vi "Create_SourceItem_from_Linker.vi"(8 "error in (no error)":errorcluster, 9 "Ignore unresolved dll reference (F)":bool, 10 "linkerInfo":T2) -> (0 "error out":errorcluster, 2 "valid?":bool, 3 "AB_Source out":refnum<class "AB_Source.lvclass">)   [LabVIEW 2020, in "AB_Source.lvclass"]
uses:
  <vilib>/AppBuilder/AB_Classes/Source/AB_Source.lvclass
  <vilib>/Utility/lvfile.llb/LVFileType.ctl
  <vilib>/AppBuilder/AB_Classes/Source/AB_Source.ctl
  <vilib>/AppBuilder/AB_Source_Inclusion.ctl
  <vilib>/AppBuilder/AB_Source_Properties.ctl
  <vilib>/AppBuilder/AB_Source_Property_Type.ctl
  <vilib>/AppBuilder/AB_Classes/Source/VI/AB_Source_VI.ctl
  <vilib>/AppBuilder/AB_Classes/Source/VI/AB_Source_VI.lvclass
  e:/builds/penguin/labview/branches/2020/dev/dist/vi.lib/AppBuilder/AB_Classes/Source/AB_Source.lvclass
  <vilib>/AppBuilder/AB_Classes/Source/Library/AB_Source_Library.ctl
  <vilib>/AppBuilder/AB_Classes/Source/Library/AB_Source_Library.lvclass
  <vilib>/AppBuilder/AB_Classes/Source/PackedItem/AB_Source_PackedItem.lvclass
  <vilib>/Utility/lvfile.llb/NI_FileType.lvlib
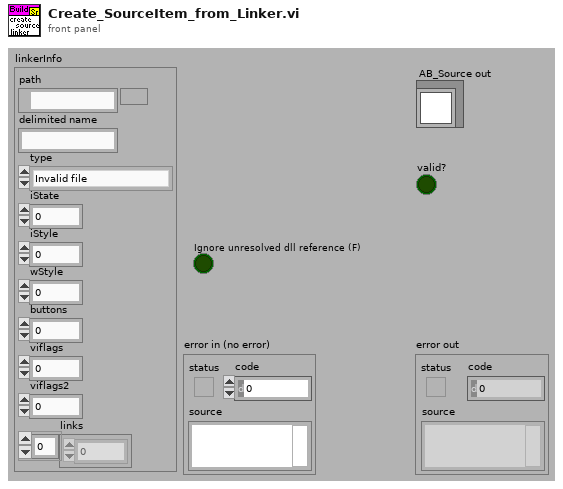
[diagram p1: front panel]
types:
  T1 = typedef "NI_FileType.lvlib/LVFileType.ctl" = enum32{"Invalid file", "Unknown type", "Instrument", "Control", "Polymorphic VI", "Project", "Library", "LVClass", "XControl", "XNode", "Shared library", ".NET assembly", "ActiveX interface", "CIN", "Run-time menu", "Palette menu", "Help file", "LLB", "XNode Edit Dependency", "Class Private Data Control", "Statechart", "MathScript .m file", "Ladder Diagram", "LVLibp", "XNode Build Dependency"}
  T2 = cluster{"path":path, "delimited name":string, "type":T1, "iState":u32, "iStyle":u16, "wStyle":u16, "buttons":u16, "viflags":u32, "viflags2":u32, "links":u32[]}
  T3 = typedef "AB_Source_VI.ctl" = cluster{"standardVI":bool, "dynamicDispatch":bool, "LLBtopLevel":bool, "privateDataControl":bool, "eng_hasNonVILinks":bool, "eng_reference":refnum<vi>, "eng_saveLevel":u32}
  T4 = typedef "AB_Source_Library.ctl" = cluster{"relinkCallers":bool, "atomicCopy":bool, "allowMissingMembers":bool, "eng_newDelimitedName":string, "eng_hasNonVILinks":bool, "eng_reference":refnum<vi>, "LVLIBPtopLevel":bool}
  T5 = typedef "AB_Source.ctl" = cluster{"path":path, "itemID":string, "parentIndex":i32, "sourceInclusion":T6, "destinationIndex":i32, "properties":T7[], "newName":string, "lvfile":bool, "valid":bool, "eng_inBuild":bool, "eng_isNonVILink":bool, "Amalgamation":bool, "Amalgamation Piece":bool, "eng_delimitedName":string, "preventRename":bool}
  T6 = typedef "AB_Source_Inclusion.ctl" = enum16{"IncludeIfReferenced", "Include", "Exclude", "TopLevel"}
  T7 = typedef "AB_Source_Properties.ctl" = cluster{"sourcePropertyType":T8, "value":variant}
  T8 = typedef "AB_Source_Property_Type.ctl" = enum16{"Remove block diagram", "Remove front panel", "Password", "Window has title bar", "Show menu bar", "Show vertical scroll bar", "Show horizontal scroll bar", "Show toolbar", "Show Abort button", "Show fp when called", "Window behavior", "Allow user to close window", "Window run-time position", "Run when opened", "Allow debugging", "Auto error handling", "Generate guard code", "Use stack variables", "Expression folding", "Integer only", "Inline subVI"}
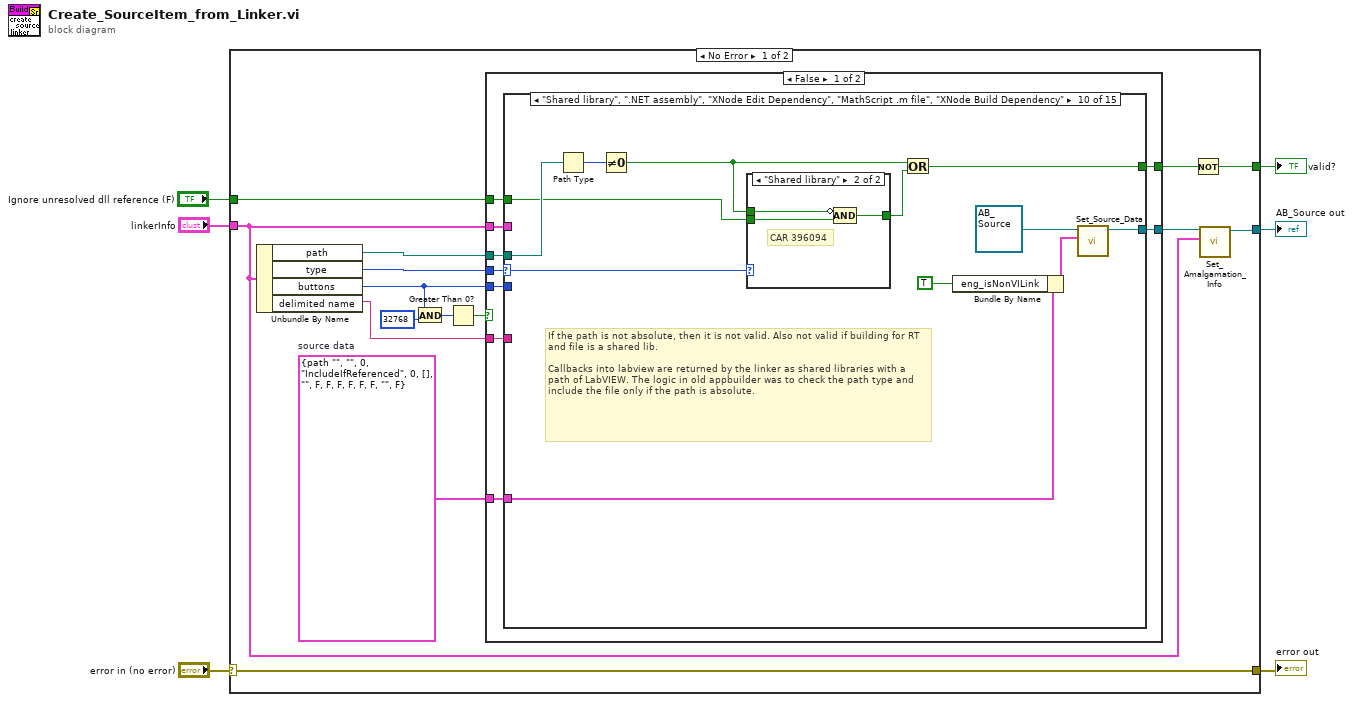
[diagram p0: block diagram]
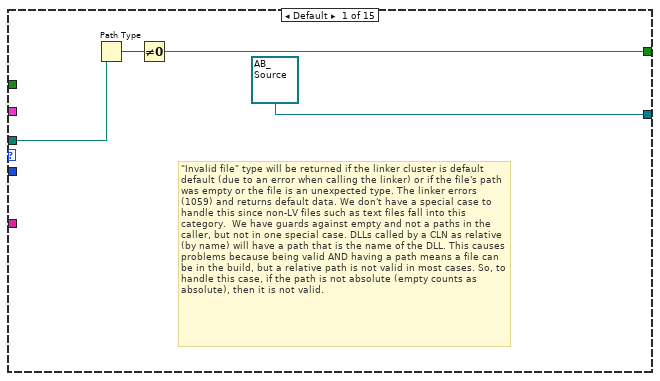
[diagram p2: hidden frame]
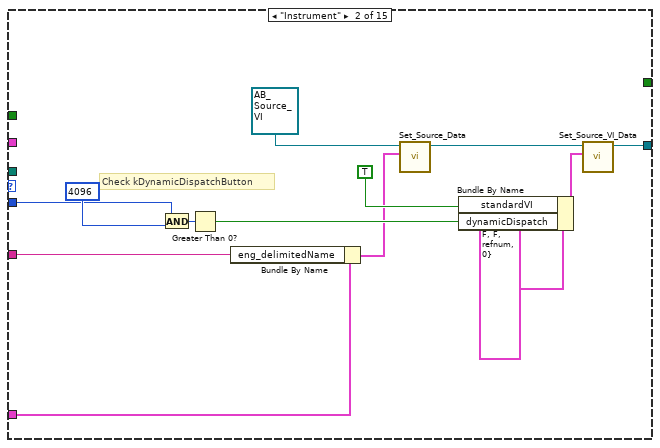
[diagram p3: hidden frame]
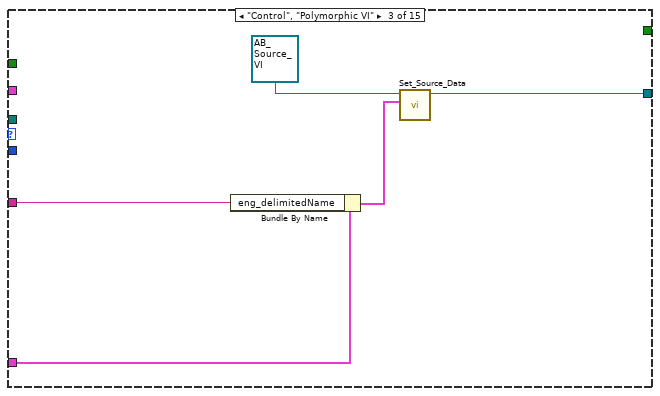
[diagram p4: hidden frame]
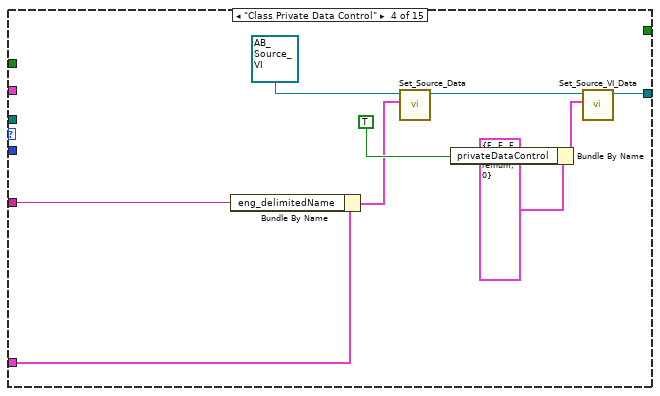
[diagram p5: hidden frame]
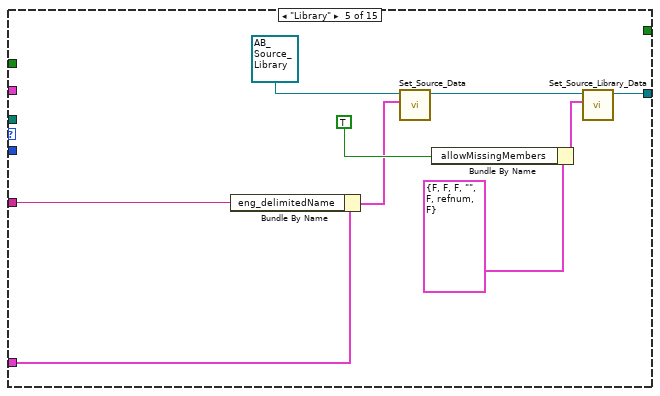
[diagram p6: hidden frame]
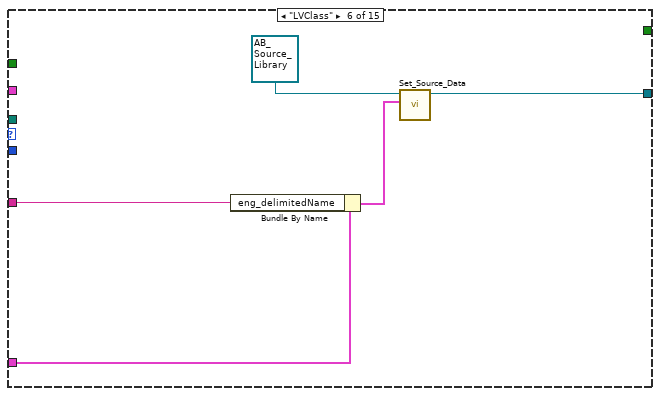
[diagram p7: hidden frame]
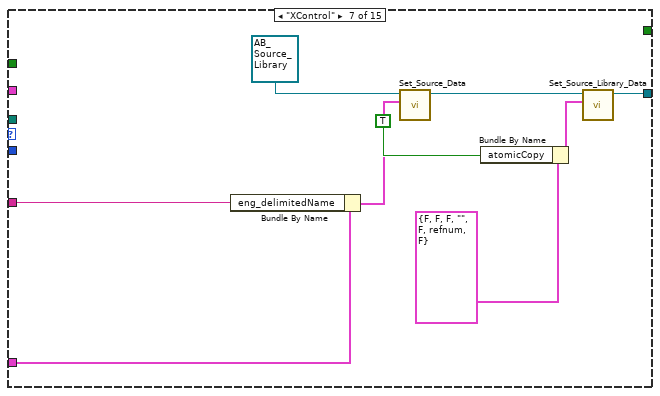
[diagram p8: hidden frame]
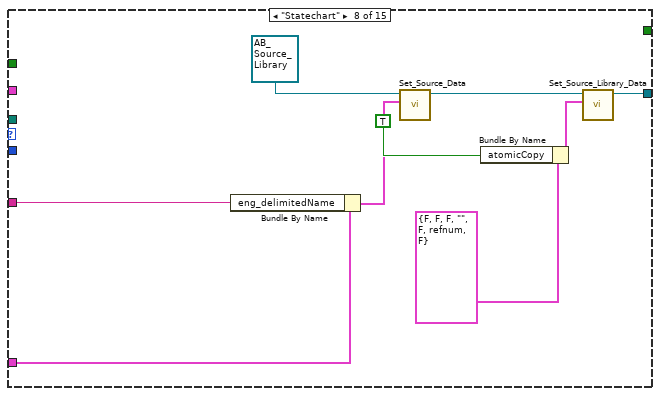
[diagram p9: hidden frame]
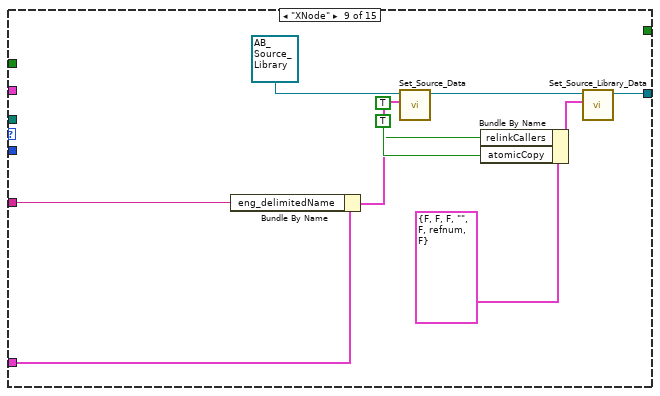
[diagram p10: hidden frame]
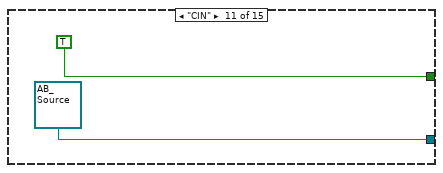
[diagram p12: hidden frame]
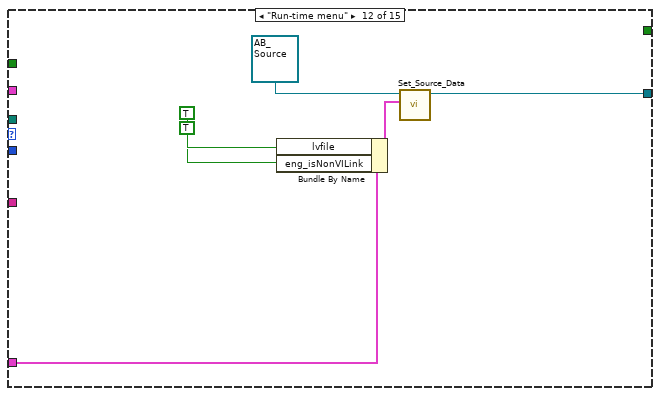
[diagram p13: hidden frame]
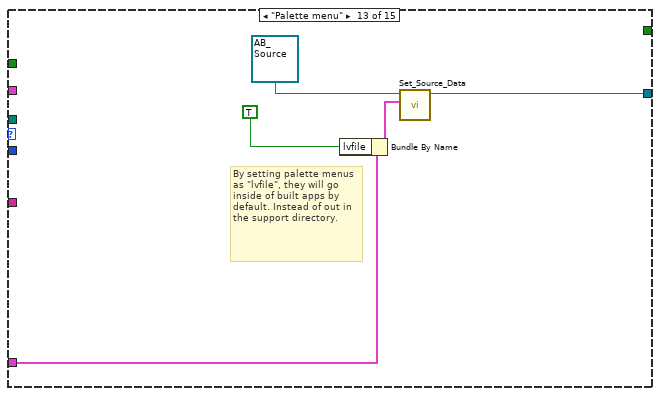
[diagram p14: hidden frame]
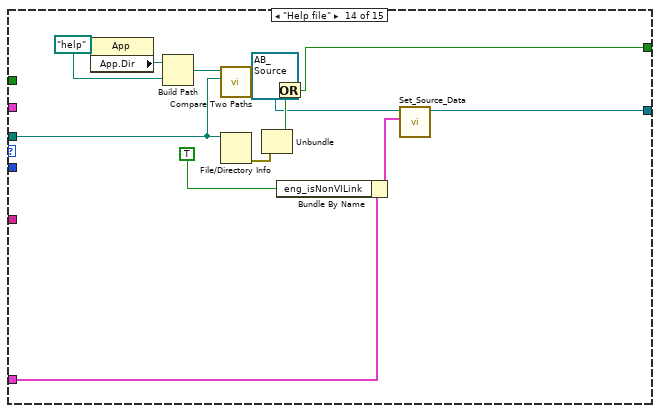
[diagram p15: hidden frame]
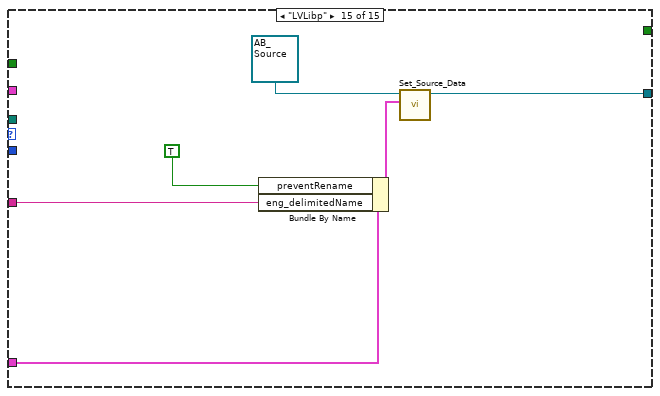
[diagram p16: hidden frame]
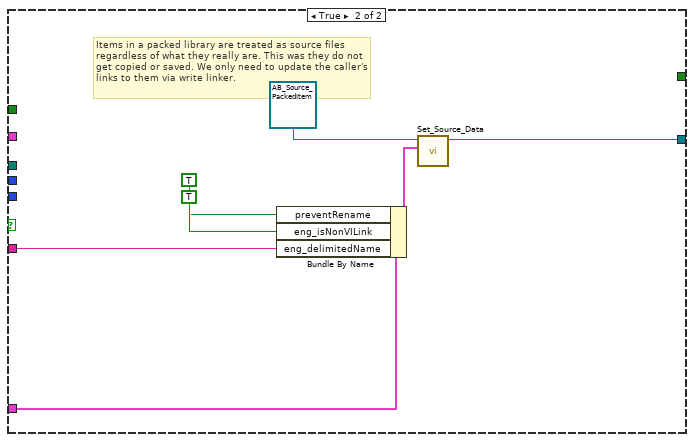
[diagram p17: hidden frame]
diagram:
  n1 = case shown="No Error" "error in (no error)" {
    selector: "error in (no error)" -> [w21 w158]
    tunnel: [w21 w158] -> w5
    tunnel: [w12 _] -> w4
    tunnel: "linkerInfo" -> [w13 _]
    tunnel: [w14 _] -> w3
    tunnel: "Ignore unresolved dll reference (F)" -> [w7 _]
    frame No Error {
      w8 = T5 {"path"=path "", "itemID"="", "parentIndex"=0, "sourceInclusion"=enum."IncludeIfReferenced", "destinationIndex"=0, "properties"=[], "newName"="", "lvfile"=FALSE, "valid"=FALSE, "eng_inBuild"=FALSE, "eng_isNonVILink"=FALSE, "Amalgamation"=FALSE, "Amalgamation Piece"=FALSE, "eng_delimitedName"="", "preventRename"=FALSE}  # source data
      n2 = Unbundle By Name(w13) -> ("path"=w18:path, "type"=w17:T1, "buttons"=w10:u16, "delimited name"=w16:string)
      n3 = And(x=w10, y=u16 32768) -> (x .and. y?=w19:u16)
      n4 = Greater Than 0?(x=w19) -> (x > 0?=w9:bool)
      n5 = case shown="False" w9 {
        tunnel: w18 -> [w30 _]
        tunnel: w17 -> [w29 _]
        tunnel: w16 -> [w28 w152]
        tunnel: [w27 _] -> w15
        tunnel: w13 -> [w26 _]
        tunnel: [w25 w154] -> w11
        tunnel: w10 -> [w24 _]
        tunnel: w8 -> [w23 w151]
        tunnel: w7 -> [w22 _]
        frame False {
          n6 = case shown="\"Shared library\", \".NET assembly\", \"XNode Edit Dependency\", \"MathScript .m file\", \"XNode Build Dependency\"" w29 {
            selector: w29 -> [_ _ _ _ _ _ _ _ _ w104 _ _ _ _ _]
            tunnel: w30 -> [w32 _ _ _ _ _ _ _ _ w115 _ _ _ w140 _]
            tunnel: w26 -> [_ _ _ _ _ _ _ _ _ _ _ _ _ _ _]
            tunnel: [w31 _ _ _ _ _ _ _ _ w107 TRUE _ _ w141 _] -> w27
            tunnel: [refnum<class "AB_Source.lvclass"> refnum ("AB_Source.lvclass") w44 w50 w60 w69 w74 w81 w90 w100 w112 refnum<class "AB_Source.lvclass"> refnum ("AB_Source.lvclass") w123 w130 w134 w148] -> w25
            tunnel: w28 -> [_ w36 w52 w54 w63 w73 w80 w89 w99 _ _ _ _ _ w145]
            tunnel: w24 -> [_ w41 _ _ _ _ _ _ _ _ _ _ _ _ _]
            tunnel: w23 -> [_ w37 w49 w55 w64 w72 w79 w88 w98 w109 _ w121 w129 w132 w146]
            tunnel: w22 -> [_ _ _ _ _ _ _ _ _ w106 _ _ _ _ _]
            frame Default {
              # "\"Invalid file\" type will be returned if the linker cluster is default default (due to an error when calling the linker) or if the file's path was empty or the file is an unexpected type. The linker errors (1059) and returns default data. We don't have a special case to handle this since non-LV files such as text files fall into this category.  We have guards against empty and not a paths in the caller, but not in one special case. DLLs called by a CLN as relative (by name) will have a path that is the name of the DLL. This causes problems because being valid AND having a path means a file can be in the build, but a relative path is not valid in most cases. So, to handle this case, if the path is not absolute (empty counts as absolute), then it is not valid."
              n7 = Path Type(1:w32) -> (0:w33:i16)
              n8 = Not Equal To 0?(x=w33) -> (x != 0?=w31:bool)
            }
            frame "Instrument" {
              # "Check kDynamicDispatchButton"
              n9 = And(x=w41, y=u16 4096) -> (x .and. y?=w43:u16)
              n10 = Greater Than 0?(x=w43) -> (x > 0?=w40:bool)
              n11 = Bundle By Name(cluster=w37, "eng_delimitedName"=w36) -> (w35:T5)
              n12 = call <vilib>:"Set_Source_Data.vi"("data"=w35, "Class in"=refnum<class "AB_Source_VI.lvclass"> refnum ("AB_Source_VI.lvclass")) -> ("Class out"=w38:refnum<class "AB_Source_VI.lvclass">)  [unwired: 8 in, 1 out]
              n13 = Bundle By Name(cluster=T3 {"standardVI"=FALSE, "dynamicDispatch"=FALSE, "LLBtopLevel"=FALSE, "privateDataControl"=FALSE, "eng_hasNonVILinks"=FALSE, "eng_reference"=refnum, "eng_saveLevel"=0} ("data"), "standardVI"=TRUE, "dynamicDispatch"=w40) -> (w45:T3)
              n14 = call <vilib>:"Set_Source_VI_Data.vi"("data"=w45, "Class in"=w38) -> ("Class out"=w44:refnum<class "AB_Source_VI.lvclass">)  [unwired: 1 in, 8 out]
            }
            frame "Control", "Polymorphic VI" {
              n15 = Bundle By Name(cluster=w49, "eng_delimitedName"=w52) -> (w48:T5)
              n16 = call <vilib>:"Set_Source_Data.vi"("data"=w48, "Class in"=refnum<class "AB_Source_VI.lvclass"> refnum ("AB_Source_VI.lvclass")) -> ("Class out"=w50:refnum<class "AB_Source_VI.lvclass">)  [unwired: 8 in, 1 out]
            }
            frame "Class Private Data Control" {
              n17 = Bundle By Name(cluster=w55, "eng_delimitedName"=w54) -> (w53:T5)
              n18 = call <vilib>:"Set_Source_Data.vi"("data"=w53, "Class in"=refnum<class "AB_Source_VI.lvclass"> refnum ("AB_Source_VI.lvclass")) -> ("Class out"=w56:refnum<class "AB_Source_VI.lvclass">)  [unwired: 8 in, 1 out]
              n19 = Bundle By Name(cluster=T3 {"standardVI"=FALSE, "dynamicDispatch"=FALSE, "LLBtopLevel"=FALSE, "privateDataControl"=FALSE, "eng_hasNonVILinks"=FALSE, "eng_reference"=refnum, "eng_saveLevel"=0} ("data"), "privateDataControl"=TRUE) -> (w59:T3)
              n20 = call <vilib>:"Set_Source_VI_Data.vi"("data"=w59, "Class in"=w56) -> ("Class out"=w60:refnum<class "AB_Source_VI.lvclass">)  [unwired: 1 in, 8 out]
            }
            frame "Library" {
              n21 = Bundle By Name(cluster=w64, "eng_delimitedName"=w63) -> (w62:T5)
              n22 = call <vilib>:"Set_Source_Data.vi"("data"=w62, "Class in"=refnum<class "AB_Source_Library.lvclass"> refnum ("AB_Source_Library.lvclass")) -> ("Class out"=w65:refnum<class "AB_Source_Library.lvclass">)  [unwired: 8 in, 1 out]
              n23 = Bundle By Name(cluster=T4 {"relinkCallers"=FALSE, "atomicCopy"=FALSE, "allowMissingMembers"=FALSE, "eng_newDelimitedName"="", "eng_hasNonVILinks"=FALSE, "eng_reference"=refnum, "LVLIBPtopLevel"=FALSE} ("data"), "allowMissingMembers"=TRUE) -> (w68:T4)
              n24 = call <vilib>:"Set_Source_Library_Data.vi"("data"=w68, "Class in"=w65) -> ("Class out"=w69:refnum<class "AB_Source_Library.lvclass">)  [unwired: 1 in, 8 out]
            }
            frame "LVClass" {
              n25 = Bundle By Name(cluster=w72, "eng_delimitedName"=w73) -> (w71:T5)
              n26 = call <vilib>:"Set_Source_Data.vi"("data"=w71, "Class in"=refnum<class "AB_Source_Library.lvclass"> refnum ("AB_Source_Library.lvclass")) -> ("Class out"=w74:refnum<class "AB_Source_Library.lvclass">)  [unwired: 8 in, 1 out]
            }
            frame "XControl" {
              n27 = Bundle By Name(cluster=w79, "eng_delimitedName"=w80) -> (w76:T5)
              n28 = call <vilib>:"Set_Source_Data.vi"("data"=w76, "Class in"=refnum<class "AB_Source_Library.lvclass"> refnum ("AB_Source_Library.lvclass")) -> ("Class out"=w77:refnum<class "AB_Source_Library.lvclass">)  [unwired: 8 in, 1 out]
              n29 = Bundle By Name(cluster=T4 {"relinkCallers"=FALSE, "atomicCopy"=FALSE, "allowMissingMembers"=FALSE, "eng_newDelimitedName"="", "eng_hasNonVILinks"=FALSE, "eng_reference"=refnum, "LVLIBPtopLevel"=FALSE} ("data"), "atomicCopy"=TRUE ("eng_includeMembers")) -> (w83:T4)
              n30 = call <vilib>:"Set_Source_Library_Data.vi"("data"=w83, "Class in"=w77) -> ("Class out"=w81:refnum<class "AB_Source_Library.lvclass">)  [unwired: 1 in, 8 out]
            }
            frame "Statechart" {
              n31 = Bundle By Name(cluster=w88, "eng_delimitedName"=w89) -> (w85:T5)
              n32 = call <vilib>:"Set_Source_Data.vi"("data"=w85, "Class in"=refnum<class "AB_Source_Library.lvclass"> refnum ("AB_Source_Library.lvclass")) -> ("Class out"=w86:refnum<class "AB_Source_Library.lvclass">)  [unwired: 8 in, 1 out]
              n33 = Bundle By Name(cluster=T4 {"relinkCallers"=FALSE, "atomicCopy"=FALSE, "allowMissingMembers"=FALSE, "eng_newDelimitedName"="", "eng_hasNonVILinks"=FALSE, "eng_reference"=refnum, "LVLIBPtopLevel"=FALSE} ("data"), "atomicCopy"=TRUE ("eng_includeMembers")) -> (w92:T4)
              n34 = call <vilib>:"Set_Source_Library_Data.vi"("data"=w92, "Class in"=w86) -> ("Class out"=w90:refnum<class "AB_Source_Library.lvclass">)  [unwired: 1 in, 8 out]
            }
            frame "XNode" {
              n35 = Bundle By Name(cluster=w98, "eng_delimitedName"=w99) -> (w95:T5)
              n36 = call <vilib>:"Set_Source_Data.vi"("data"=w95, "Class in"=refnum<class "AB_Source_Library.lvclass"> refnum ("AB_Source_Library.lvclass")) -> ("Class out"=w96:refnum<class "AB_Source_Library.lvclass">)  [unwired: 8 in, 1 out]
              n37 = Bundle By Name(cluster=T4 {"relinkCallers"=FALSE, "atomicCopy"=FALSE, "allowMissingMembers"=FALSE, "eng_newDelimitedName"="", "eng_hasNonVILinks"=FALSE, "eng_reference"=refnum, "LVLIBPtopLevel"=FALSE} ("data"), "relinkCallers"=TRUE, "atomicCopy"=TRUE ("eng_includeMembers")) -> (w102:T4)
              n38 = call <vilib>:"Set_Source_Library_Data.vi"("data"=w102, "Class in"=w96) -> ("Class out"=w100:refnum<class "AB_Source_Library.lvclass">)  [unwired: 1 in, 8 out]
            }
            frame "Shared library", ".NET assembly", "XNode Edit Dependency", "MathScript .m file", "XNode Build Dependency" {
              # "If the path is not absolute, then it is not valid. Also not valid if building for RT and file is a shared lib.\n\nCallbacks into labview are returned by the linker as shared libraries with a path of LabVIEW. The logic in old appbuilder was to check the path type and include the file only if the path is absolute."
              n39 = Path Type(1:w115) -> (0:w114:i16)
              n40 = Not Equal To 0?(x=w114) -> (x != 0?=w105:bool)
              n41 = case shown="\"Shared library\"" w104 {
                tunnel: [_ w118] -> w108
                tunnel: w106 -> [_ w117]
                tunnel: w105 -> [_ w116]
                frame Default {
                }
                frame "Shared library" {
                  # "CAR 396094"
                  n42 = Compound Arithmetic op=AND(invert w116, w117) -> (w118:bool)
                }
              }
              n43 = Or(x=w105, y=w108) -> (x .or. y?=w107:bool)
              n44 = Bundle By Name(cluster=w109, "eng_isNonVILink"=TRUE) -> (w110:T5)
              n45 = call <vilib>:"Set_Source_Data.vi"("data"=w110, "Class in"=refnum<class "AB_Source.lvclass"> refnum ("AB_Source.lvclass")) -> ("Class out"=w112:refnum<class "AB_Source.lvclass">)  [unwired: 1 in, 8 out]
            }
            frame "CIN" {
            }
            frame "Run-time menu" {
              n46 = Bundle By Name(cluster=w121, "lvfile"=TRUE ("eng_isNonVILink"), "eng_isNonVILink"=TRUE) -> (w124:T5)
              n47 = call <vilib>:"Set_Source_Data.vi"("data"=w124, "Class in"=refnum<class "AB_Source.lvclass"> refnum ("AB_Source.lvclass")) -> ("Class out"=w123:refnum<class "AB_Source.lvclass">)  [unwired: 1 in, 8 out]
            }
            frame "Palette menu" {
              # "By setting palette menus as \"lvfile\", they will go inside of built apps by default. Instead of out in the support directory."
              n48 = Bundle By Name(cluster=w129, "lvfile"=TRUE ("eng_isNonVILink")) -> (w128:T5)
              n49 = call <vilib>:"Set_Source_Data.vi"("data"=w128, "Class in"=refnum<class "AB_Source.lvclass"> refnum ("AB_Source.lvclass")) -> ("Class out"=w130:refnum<class "AB_Source.lvclass">)  [unwired: 1 in, 8 out]
            }
            frame "Help file" {
              n50 = property class="App"() -> ("App.Dir"=w138:path)  [unwired: 2 in, 2 out]
              n51 = Build Path(base path=w138, name or relative path=path "help" ("Application:Directory Path")) -> (appended path=w137:path)
              n52 = call <vilib>:"Compare Two Paths.vi"("Path 2"=w140, "Path 1"=w137) -> ("Path 2 Relative to Path 1?"=w143:bool)  [unwired: 1 in, 8 out]
              n53 = File/Directory Info(path=w140) -> (error out=w144:errorcluster)  [unwired: 1 in, 6 out]
              n54 = Unbundle(w144) -> ("status"=w142:bool)  [unwired: 2 out]
              n55 = Or(x=w143, y=w142) -> (x .or. y?=w141:bool)
              n56 = Bundle By Name(cluster=w132, "eng_isNonVILink"=TRUE) -> (w135:T5)
              n57 = call <vilib>:"Set_Source_Data.vi"("data"=w135, "Class in"=refnum<class "AB_Source.lvclass"> refnum ("AB_Source.lvclass")) -> ("Class out"=w134:refnum<class "AB_Source.lvclass">)  [unwired: 1 in, 8 out]
            }
            frame "LVLibp" {
              n58 = Bundle By Name(cluster=w146, "preventRename"=TRUE ("eng_preventRename"), "eng_delimitedName"=w145) -> (w149:T5)
              n59 = call <vilib>:"Set_Source_Data.vi"("data"=w149, "Class in"=refnum<class "AB_Source.lvclass"> refnum ("AB_Source.lvclass")) -> ("Class out"=w148:refnum<class "AB_Source.lvclass">)  [unwired: 1 in, 8 out]
            }
          }
        }
        frame True {
          # "Items in a packed library are treated as source files regardless of what they really are. This was they do not get copied or saved. We only need to update the caller's links to them via write linker."
          n60 = Bundle By Name(cluster=w151, "preventRename"=TRUE ("eng_preventRename"), "eng_isNonVILink"=TRUE, "eng_delimitedName"=w152) -> (w155:T5)
          n61 = call <vilib>:"Set_Source_Data.vi"("data"=w155, "Class in"=refnum<class "AB_Source_PackedItem.lvclass"> refnum ("AB_Source_PackedItem.lvclass")) -> ("Class out"=w154:refnum<class "AB_Source_PackedItem.lvclass">)  [unwired: 1 in, 8 out]
        }
      }
      n62 = Not(x=w15) -> (.not. x?=w14:bool)
      n63 = call <vilib>:"Set_Amalgamation_Info.vi"("linkerInfo"=w13, "Source In"=w11) -> ("Source Out"=w12:refnum<class "AB_Source.lvclass">)  [unwired: 9 out]
    }
    frame Error {
    }
  }
  "error out" <- w5
  "AB_Source out" <- w4
  "valid?" <- w3
